vi "CheckIfSubpanel.vi"(8 "error in":errorcluster, 11 "Object Layout in":refnum<class "Object Layout.lvclass">) -> (0 "error out":errorcluster, 2 "subpanel?":bool, 3 "Object Layout out":refnum<class "Object Layout.lvclass">)   [LabVIEW 2010, in "NI_SE_Front Panel Layout.lvlib" / "Object Layout.lvclass"]
uses:
  Object Layout.lvclass
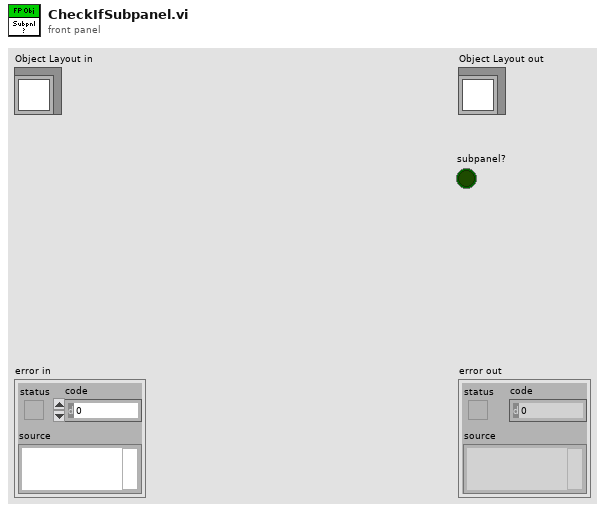
[diagram p1: front panel]
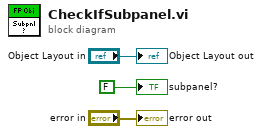
[diagram p0: block diagram]
diagram:
  "error out" <- "error in"
  "Object Layout out" <- "Object Layout in"
  "subpanel?" <- FALSE ("Boolean")
